vi "Poll.InitializeTree.vi"(8 "error in (no error)":errorcluster, 9 "Refs":T1[](array[typedef]) format="%.0x", 10 "Node Pointer":T2, 11 "TreeBrowserRef":refnum<k24>) -> (0 "error out":errorcluster, 2 "Channels":variant, 3 "TreeBrowserRef 2":refnum<k24>)   [LabVIEW 2019, in "OPC UA Client Addon System Explorer.lvlib"]
uses:
  OPC UA Client Addon System Explorer.lvlib
  <vilib>/NI VeriStand/Custom Device API/Custom Device Pointer.ctl
  NationalInstruments.VeriStand.SystemStorage
  NationalInstruments.VeriStand.SystemStorageUI
  <vilib>/NI VeriStand/Custom Device API/Custom Device Item Ref.ctl
  NationalInstruments.VeriStand
  Addon Shared/Constants.vi
  <vilib>/NI VeriStand/Custom Device API/Custom Device API.lvlib
  Addon Shared/OPC UA Client Addon Shared.lvlib
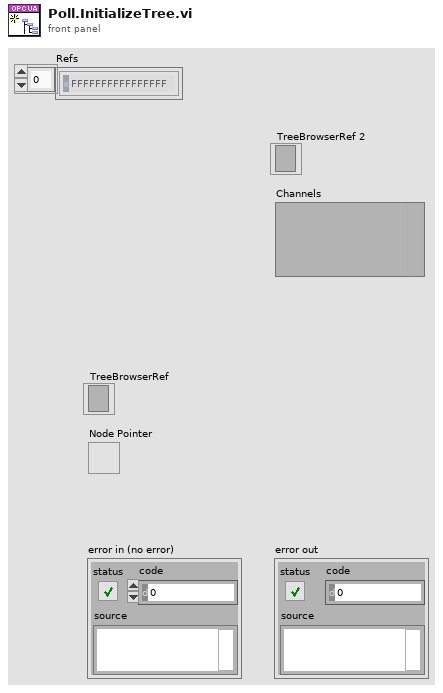
[diagram p1: front panel]
types:
  T1 = typedef "Custom Device API.lvlib/Custom Device Item Ref.ctl" = u64
  T2 = typedef "Custom Device API.lvlib/Custom Device Pointer.ctl" = refnum<k24>
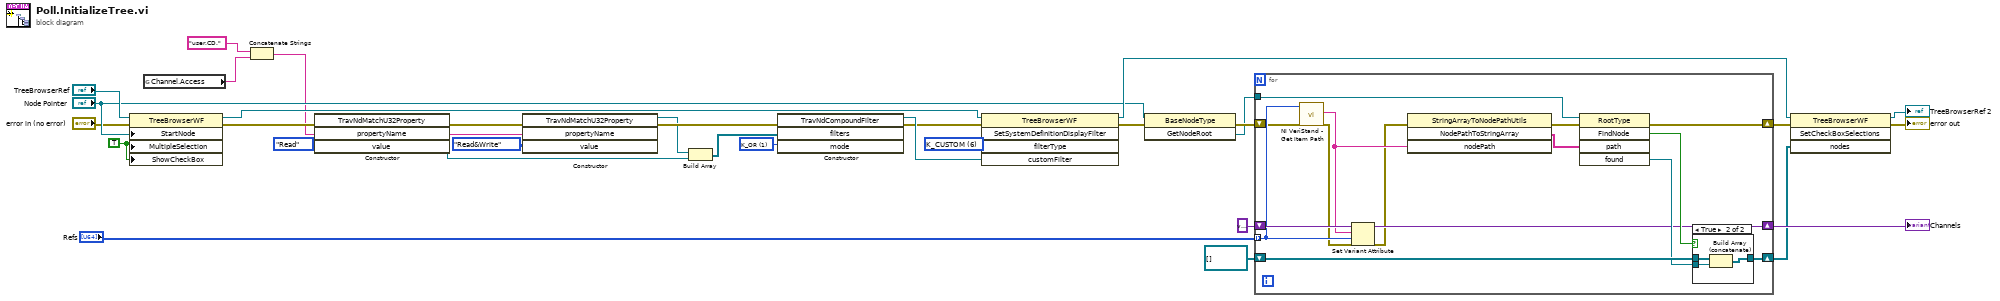
[diagram p0: block diagram]
diagram:
  w14 = 1 items=["K_AND", "K_OR"] ("mode")
  w26 = TRUE ("MultipleSelection")
  w18 = u8 6 items=["K_CHAN_R", "K_CHAN_W", "K_CHAN_RW", "K_CHAN_VOLT", "K_CHAN_FAULT", "K_ALL", "K_CUSTOM", "K_CHAN_R_VIS", "K_CHAN_W_VIS", "K_CHAN_RW_VIS", "K_CHAN_VOLT_VIS", "K_CHAN_FAULT_VIS", "K_WAVE", "K_WAVE_VIS", "K_WAVE_DBL", "K_WAVE_CDB", "K_WAVE_DBL_VIS", "K_WAVE_CDB_VIS"] ("filterType")
  n1 = property class="TreeBrowserWF"(reference="TreeBrowserRef", error in="error in (no error)", "StartNode"="Node Pointer", "MultipleSelection"=w26, "ShowCheckBox"=w26) -> (reference out=w20:refnum<k24>, error out=w7:errorcluster)
  n2 = global read "Constants.vi" "Channel.Access"() -> (w2:string)
  n3 = Concatenate Strings("user.CD." ("string"), w2) -> (w1:string)
  n4 = constructor class="TravNdMatchU32Property"(error in=w7, "propertyName"=w1, "value"=enum16{"Null", "Read", "Write", "Read&Write"}."Read" ("access")) -> (reference out=w4:refnum<k24>, error out=w8:errorcluster)  [unwired: 2 in, 3 out]
  n5 = constructor class="TravNdMatchU32Property"(error in=w8, "propertyName"=w1, "value"=enum16{"Null", "Read", "Write", "Read&Write"}."Read&Write" ("access")) -> (reference out=w5:refnum<k24>, error out=w6:errorcluster)  [unwired: 2 in, 3 out]
  n6 = Build Array(w5, w4) -> (w11:refnum<k24>[])
  n7 = constructor class="TravNdCompoundFilter"(error in=w6, "filters"=w11, "mode"=w14) -> (reference out=w13:refnum<k24>, error out=w12:errorcluster)  [unwired: 2 in, 3 out]
  n8 = invoke class="TreeBrowserWF" method="SetSystemDefinitionDisplayFilter"(reference=w20, error in=w12, "filterType"=w18, "customFilter"=w13) -> (reference out=w22:refnum<k24>, error out=w31:errorcluster)  [unwired: 1 in, 3 out]
  n9 = invoke class="BaseNodeType" method="GetNodeRoot"(reference="Node Pointer", error in=w31) -> (error out=w32:errorcluster, "GetNodeRoot"=w30:refnum<k24>)  [unwired: 1 in, 1 out]
  n10 = for {
    shift-right: [w44] -> w25
    shift-left: w32 -> [w36]
    tunnel: "Refs" -> [w37] mode=indexing
    tunnel: w30 -> [w47]
    shift-right: [w41] -> w27
    shift-left: refnum<k24>[] [] -> [w42]
    shift-right: [w38] -> w29
    shift-left: variant -> [w39]
    n11 = call <vilib>:"NI VeriStand - Get Item Path.vi"("error in (no error)"=w36, "Item Ref in"=w37) -> ("error out"=w34:errorcluster, "Path"=w35:string)  [unwired: 6 in, 2 out]
    n12 = Set Variant Attribute(Variant=w39, name=w35, value=w37, error in=w34) -> (Variant out=w38:variant, error out=w33:errorcluster)  [unwired: 1 out]
    n13 = invoke class="StringArrayToNodePathUtils" method="NodePathToStringArray"(error in=w33, "nodePath"=w35) -> (error out=w45:errorcluster, "NodePathToStringArray"=w46:string[])  [unwired: 2 in, 2 out]
    n14 = invoke class="RootType" method="FindNode"(reference=w47, error in=w45, "path"=w46) -> (error out=w44:errorcluster, "FindNode"=w43:bool, "found"=w40:refnum<k24>)  [unwired: 2 in, 2 out]
    n15 = case shown="True" w43 {
      tunnel: w42 -> [w48 w51]
      tunnel: [w48 w49] -> w41
      tunnel: w40 -> [_ w50]
      frame False {
      }
      frame True {
        n16 = Build Array (concatenate)(w51, w50) -> (w49:refnum<k24>[])
      }
    }
  }
  "Channels" <- w29
  n17 = invoke class="TreeBrowserWF" method="SetCheckBoxSelections"(reference=w22, error in=w25, "nodes"=w27) -> (reference out=→"TreeBrowserRef 2":refnum<k24>, error out=→"error out":errorcluster)  [unwired: 1 in, 2 out]
